vi "Get Port Status.vi"(8 "error in (no error)":errorcluster, 10 "Puerto":string, 11 "UI Actor in":refnum<class "UI Actor.lvclass">) -> (0 "error out":errorcluster, 3 "UI Actor out":refnum<class "UI Actor.lvclass">)   [LabVIEW 2020, in "UI Actor.lvlib" / "UI Actor.lvclass"]
doc: "Obtiene el valor del puerto del micro de la marca seleccionado"
uses:
  UI Actor.lvclass
  UI Actor.lvclass/UI Actor.ctl
  Abstract/Serial Device/Serial Device.lvclass
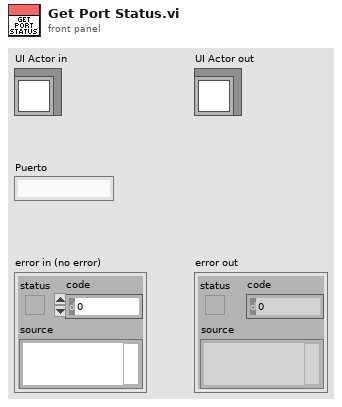
[diagram p1: front panel]
types:
  T1 = typedef "Control 1.ctl" = string
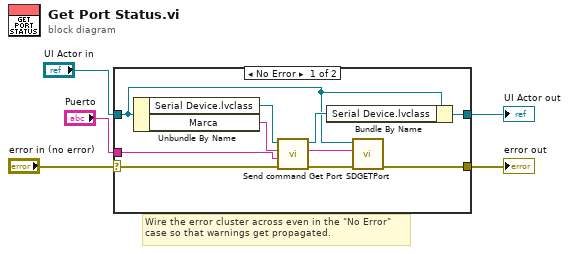
[diagram p0: block diagram]
diagram:
  # "Wire the error cluster across even in the \"No Error\"\ncase so that warnings get propagated."
  n1 = case shown="No Error" "error in (no error)" {
    selector: "error in (no error)" -> [w12 w17]
    tunnel: [w7 w17] -> w4
    tunnel: [w14 w16] -> w2
    tunnel: "UI Actor in" -> [w9 w16]
    tunnel: "Puerto" -> [w10 _]
    frame No Error {
      n2 = Unbundle By Name(w9) -> ("Serial Device.lvclass"=w15:refnum<class "Serial Device.lvclass">, "Marca"=w11:T1)
      n3 = call-dynamic "Send command Get Port.vi"("error in (no error)"=w12, "Puerto"=w10, "Marca"=w11, "Serial Device in"=w15) -> ("error out"=w8:errorcluster, "Expected response"=w6:string, "Serial Device out"=w13:refnum<class "Serial Device.lvclass">)  [unwired: 4 in, 1 out]
      n4 = Bundle By Name(cluster=w9, "Serial Device.lvclass"=w13) -> (w14:refnum<class "UI Actor.lvclass">)
      n5 = call "SDGETPort.vi"("error in (no error)"=w8, "Expected response"=w6, "UI Actor in"=w9) -> ("error out"=w7:errorcluster)  [unwired: 8 in]
    }
    frame Error {
    }
  }
  "error out" <- w4
  "UI Actor out" <- w2
